vi "FestoCPX.Station.Prod.Take.vi"(8 "error in":errorcluster, 10 "SuckerID":i32, 11 "Slot":T1) -> (0 "error out":errorcluster)   [LabVIEW 2016]
uses:
  Station/Station.ProductSlot.ctl
  Station/Station.ValvePosition.ctl
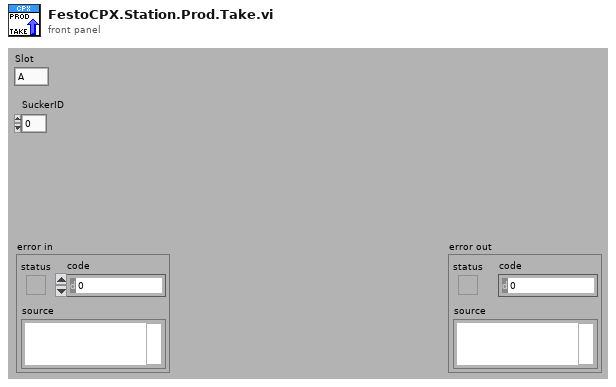
[diagram p1: front panel]
types:
  T1 = typedef "Station.ProductSlot.ctl" = enum8{"A", "B"}
  T2 = typedef "Station.ValvePosition.ctl" = enum16{"Home", "Work"}
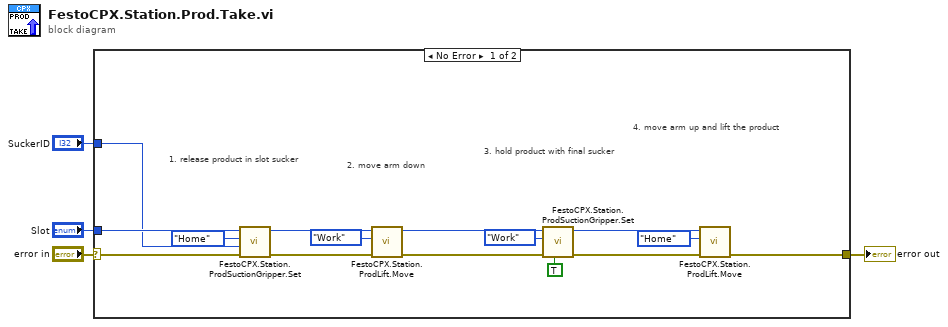
[diagram p0: block diagram]
diagram:
  n1 = case shown="No Error" "error in" {
    selector: "error in" -> [w5 w17]
    tunnel: [w16 w17] -> w4
    tunnel: "Slot" -> [w15 _]
    tunnel: "SuckerID" -> [w14 _]
    frame No Error {
      # "2. move arm down"
      # "4. move arm up and lift the product"
      # "3. hold product with final sucker"
      # "1. release product in slot sucker"
      n2 = call "FestoCPX.Station.ProdSuctionGripper.Set.vi"("error in"=w5, "Sucker (0: Final)"=w14, "Position"=Station.ValvePosition."Home", "Slot"=w15) -> ("error out"=w6:errorcluster)  [unwired: 6 in, 1 out]
      n3 = call "FestoCPX.Station.ProdLift.Move.vi"("error in"=w6, "Position"=Station.ValvePosition."Work", "Slot"=w15) -> ("error out"=w7:errorcluster)  [unwired: 8 in]
      n4 = call "FestoCPX.Station.ProdSuctionGripper.Set.vi"("wait for product (F)"=TRUE, "error in"=w7, "Position"=Station.ValvePosition."Work", "Slot"=w15) -> ("error out"=w11:errorcluster)  [unwired: 6 in, 1 out]
      n5 = call "FestoCPX.Station.ProdLift.Move.vi"("error in"=w11, "Position"=Station.ValvePosition."Home", "Slot"=w15) -> ("error out"=w16:errorcluster)  [unwired: 8 in]
    }
    frame Error {
    }
  }
  "error out" <- w4
